vi "UploadSerialNumber.vi"(8 "error in (no error)":errorcluster, 10 "UploadSerialNumber":cluster{"Socket":i32, "SerialNumber":string}, 11 "TestBench in":refnum<class "TestBench.lvclass">) -> (0 "error out":errorcluster, 3 "TestBench out":refnum<class "TestBench.lvclass">)   [LabVIEW 2019, in "TestBench.lvlib" / "TestBench.lvclass"]
uses:
  TestBench.lvclass
  TestBench.lvclass/TestBench.ctl
  TestEngine/TestEngine Messages/Write SerialNumber Msg/Write SerialNumber Msg.lvclass/Write SerialNumber Msg.ctl
  <vilib>/ActorFramework/Message Enqueuer/Message Enqueuer.lvclass/Message Enqueuer.ctl
  <vilib>/ActorFramework/Message Enqueuer/Enqueue.vi
  TestEngine/TestEngine Messages/Write SerialNumber Msg/Write SerialNumber Msg.lvclass
  C:/Program Files (x86)/National Instruments/LabVIEW 2019/vi.lib/ActorFramework/Message/Message.lvclass
  <vilib>/ActorFramework/Message Priority Queue/Priority Enqueue.vi
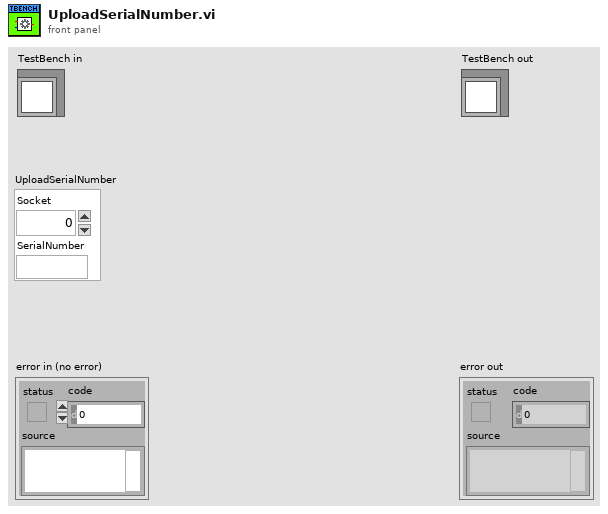
[diagram p1: front panel]
types:
  T1 = map{string, refnum<class "Message Enqueuer.lvclass">}
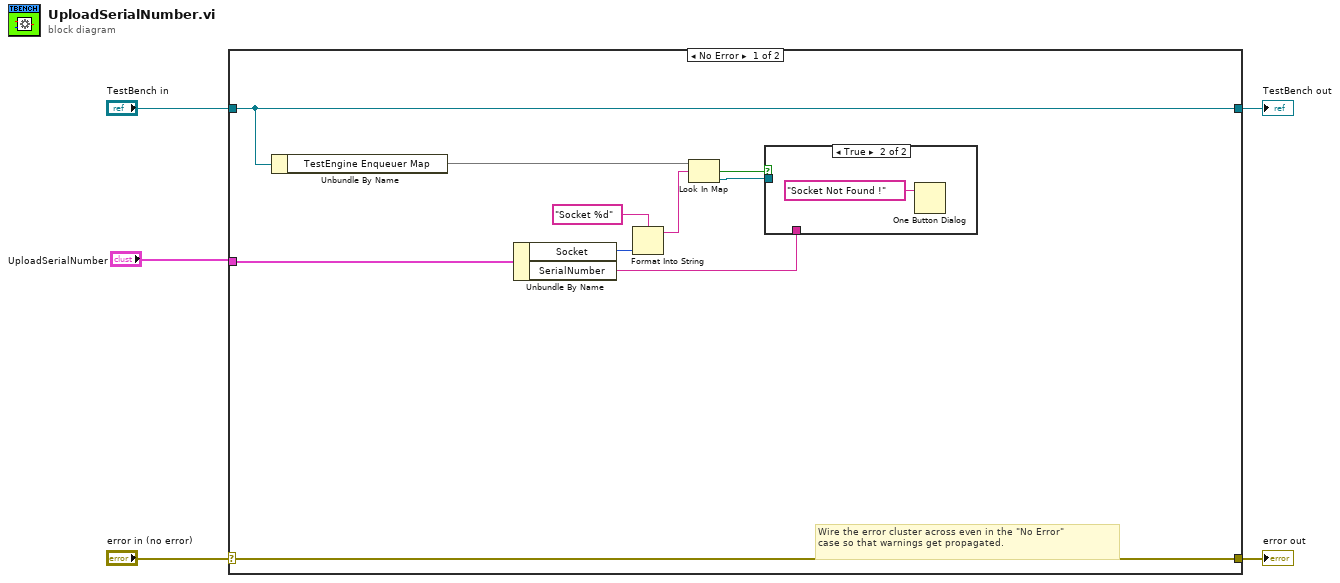
[diagram p0: block diagram]
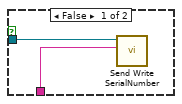
[diagram p2: hidden frame]
diagram:
  n1 = case shown="No Error" "error in (no error)" {
    selector: "error in (no error)" -> [w15 w20]
    tunnel: [w15 w20] -> w4
    tunnel: [w11 w19] -> w2
    tunnel: "TestBench in" -> [w11 w19]
    tunnel: "UploadSerialNumber" -> [w10 _]
    frame No Error {
      # "Wire the error cluster across even in the \"No Error\"\ncase so that warnings get propagated."
      n2 = Unbundle By Name(w11) -> ("TestEngine Enqueuer Map"=w9:T1)
      n3 = Unbundle By Name(w10) -> ("Socket"=w13:i32, "SerialNumber"=w7:string)
      n4 = Format Into String(format string="Socket %d", w13) -> (resulting string=w12:string)  [unwired: 2 in, 1 out]
      n5 = Look In Map(map=w9, key=w12) -> (key not found?=w6:bool, value=w8:refnum<class "Message Enqueuer.lvclass">)  [unwired: 1 in]
      n6 = case shown="True" w6 {
        tunnel: w8 -> [w17 _]
        tunnel: w7 -> [w16 _]
        frame False {
          n7 = call "Send Write SerialNumber.vi"("SerialNumber"=w16, "Message Enqueuer"=w17) -> ()  [unwired: 8 in, 2 out]
        }
        frame True {
          n8 = One Button Dialog(message="Socket Not Found !") -> ()  [unwired: 1 in, 1 out]
        }
      }
    }
    frame Error {
    }
  }
  "error out" <- w4
  "TestBench out" <- w2
